vi "Counter Page.vi"(8 "error in (no error)":errorcluster, 11 "Node Ptr":T1 format="%.0x") -> (0 "error out":errorcluster)   [LabVIEW 2020, in "Protection and Counter Addon System Explorer.lvlib"]
uses:
  Protection and Counter Addon System Explorer.lvlib
  <vilib>/NI VeriStand/Custom Device API/Custom Device Item Ref.ctl
  Addon Shared/SubVIs/GUID Lookup.vi
  <vilib>/NI VeriStand/Custom Device API/Custom Device API.lvlib
  SubModules/Frame-Protection-Support/Source/System Explorer/Protection and Counter Support System Explorer.lvlib
  Addon Shared/Protection and Counter Addon Shared.lvlib
panel:
  in  "SHDocVw.IWebBrowser":refnum<k7>(container)
  in  "Rolling Counter Max Count":dbl
  in  "Header":cluster{"Section Name":string}={"Section Name"="Counter Settings"}
  in  "Description":string
  out "Name":string
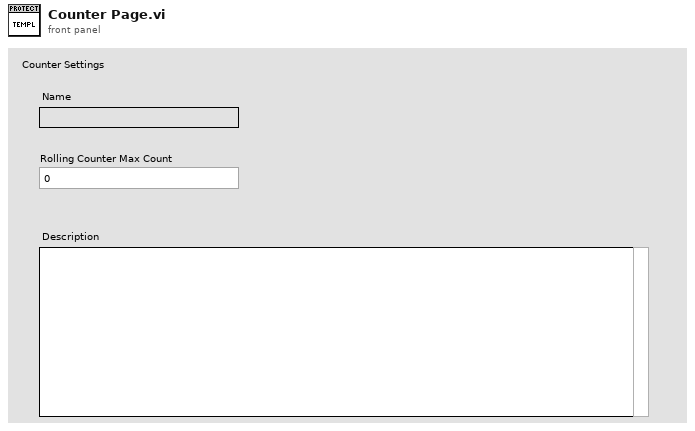
[diagram p1: front panel]
types:
  T1 = typedef "Custom Device API.lvlib/Custom Device Item Ref.ctl" = u64
  T2 = typedef "Custom Device API.lvlib/Custom Device Item Info.ctl" = cluster{"Name":string, "Is Channel":bool, "GUID":string, "Is Waveform":bool}
  T3 = typedef "Custom Device API.lvlib/Custom Device Commands.ctl" = enum16{"Default", "Item renamed", "Shutdown", "Dynamic button pressed"}
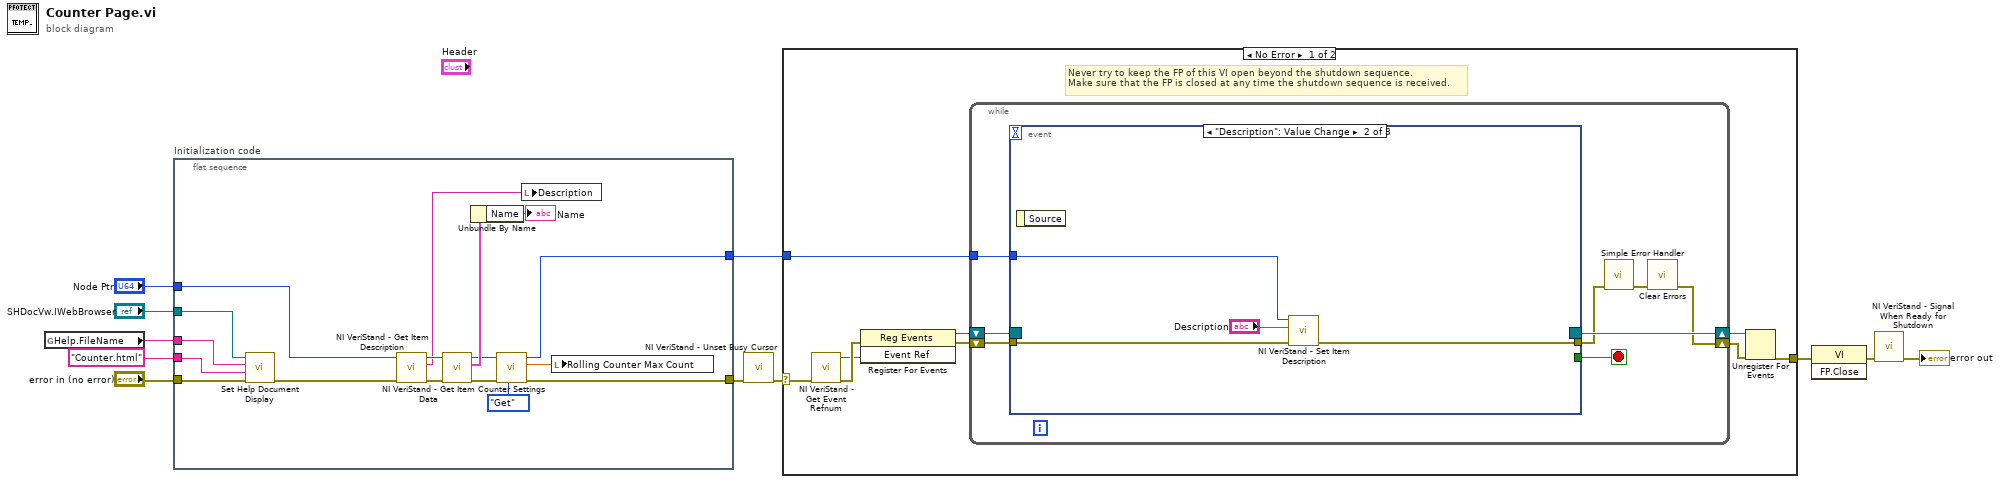
[diagram p0: block diagram]
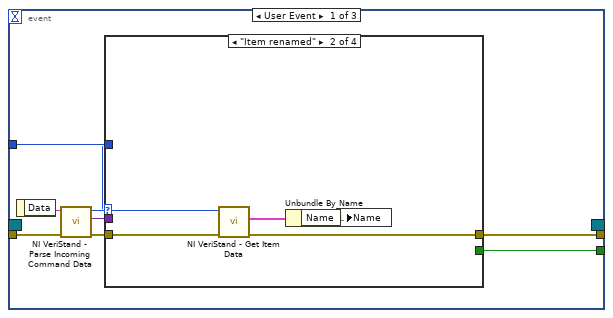
[diagram p2: hidden frame]
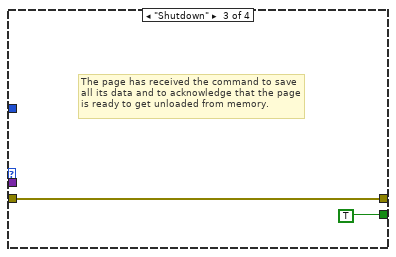
[diagram p4: hidden frame]
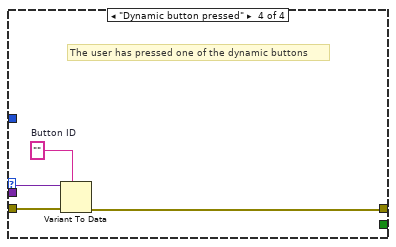
[diagram p5: hidden frame]
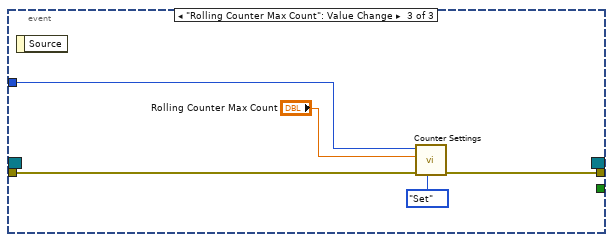
[diagram p6: hidden frame]
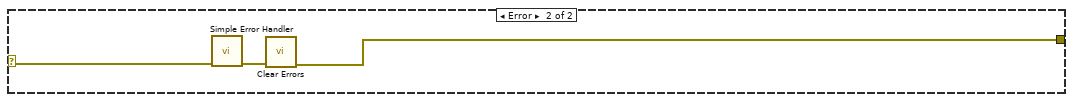
[diagram p7: hidden frame]
diagram:
  n1 = global read "GUID Lookup.vi" "Help.FileName"() -> (w1:string)
  n2 = flat-sequence "Initialization code" {
    tunnel: "error in (no error)" -> [w17]
    tunnel: "Node Ptr" -> [w27]
    tunnel: [w22] -> w7
    tunnel: [w19] -> w4
    tunnel: "Counter.html" ("HTML File") -> [w15]
    tunnel: w1 -> [w14]
    tunnel: "SHDocVw.IWebBrowser" -> [w13]
    frame #0 {
      n3 = call "Set Help Document Display.vi"("error in (no error)"=w17, "HTML File"=w15, "Main CHM File"=w14, "SHDocVw.IWebBrowser2"=w13) -> ("error out"=w16:errorcluster)  [unwired: 7 in]
      n4 = call <vilib>:"NI VeriStand - Get Item Description.vi"("error in (no error)"=w16, "Item Ref in"=w27) -> ("error out"=w25:errorcluster, "Description"=w26:string, "Item Ref out"=w28:T1)  [unwired: 7 out]
      n5 = call <vilib>:"NI VeriStand - Get Item Data.vi"("error in (no error)"=w25, "Item Ref in"=w28) -> ("error out"=w20:errorcluster, "Item Info"=w24:T2, "Item Ref out"=w18:T1)  [unwired: 7 out]
      n6 = Unbundle By Name(w24) -> ("Name"=→"Name":string)
      n7 = call "Counter Settings.vi"("Action"=enum8{"Get", "Set"}."Get", "error in"=w20, "Parent Ref"=w18) -> ("error out"=w22:errorcluster, "Max Count"=w21:dbl, "Parent Ref Out"=w19:T1)  [unwired: 6 in]
      n8 = local write "Description"(w26) -> ()
      n9 = local write "Rolling Counter Max Count"(w21) -> ()
    }
  }
  n10 = call <vilib>:"NI VeriStand - Unset Busy Cursor.vi"("error in (no error)"=w7) -> ("error out"=w6:errorcluster)  [unwired: 10 out]
  n11 = case shown="No Error" w6 {
    selector: w6 -> [w29 w77]
    tunnel: [w34 w75] -> w11
    tunnel: w4 -> [w30 _]
    frame No Error {
      # "Never try to keep the FP of this VI open beyond the shutdown sequence.\nMake sure that the FP is closed at any time the shutdown sequence is received."
      n12 = call <vilib>:"NI VeriStand - Get Event Refnum.vi"("error in (no error)"=w29) -> ("error out"=w37:errorcluster, "Event Ref"=w33:refnum<user-event>)  [unwired: 9 out]
      n13 = register-events(error in=w37, w33) -> (reference out=w31:refnum<event-registration>, error out=w32:errorcluster)  [unwired: 1 in]
      n14 = while {
        tunnel: w30 -> [w41]
        shift-right: [w38] -> w35
        shift-left: w32 -> [w44]
        shift-right: [w45] -> w36
        shift-left: w31 -> [w43]
        stop <- w42 stop-if-true
        n15 = event shown="[1] \"Description\": Value Change" {
          selector: w43 -> [_ _ _]
          dyn-events: [_ _ _] -> w45
          timeout: _ -> [_ _ _]
          tunnel: w44 -> [w53 w68 w74]
          tunnel: [w49 _ _] -> w42
          tunnel: [w48 w67 w72] -> w40
          tunnel: w41 -> [w47 w69 w73]
          event User Event {
            n16 = event-data() -> ("Data"=w52:string)  [unwired: 1 out]
            n17 = call <vilib>:"NI VeriStand - Parse Incoming Command Data.vi"("error in (no error)"=w53, "Incoming data"=w52) -> ("error out"=w51:errorcluster, "Outgoing data"=w46:variant, "Action"=w50:T3)  [unwired: 7 out]
            n18 = case shown="\"Item renamed\"" w50 {
              tunnel: w51 -> [w54 w59 w60 w65]
              tunnel: [_ _ TRUE _] -> w49
              tunnel: [w54 w56 w60 w62] -> w48
              tunnel: w47 -> [_ w58 _ _]
              tunnel: w46 -> [_ _ _ w64]
              frame "Default", Default {
              }
              frame "Item renamed" {
                n19 = call <vilib>:"NI VeriStand - Get Item Data.vi"("error in (no error)"=w59, "Item Ref in"=w58) -> ("error out"=w56:errorcluster, "Item Info"=w57:T2)  [unwired: 8 out]
                n20 = Unbundle By Name(w57) -> ("Name"=w55:string)
                n21 = local write "Name"(w55) -> ()
              }
              frame "Shutdown" {
                # "The page has received the command to save all its data and to acknowledge that the page is ready to get unloaded from memory."
              }
              frame "Dynamic button pressed" {
                w63 = ""  # Button ID
                # "The user has pressed one of the dynamic buttons"
                n22 = Variant To Data(error in=w65, type=w63, Variant=w64) -> (error out=w62:errorcluster)  [unwired: 1 out]
              }
            }
          }
          event "Description": Value Change {
            n23 = event-data() -> ()  [unwired: 2 out]
            n24 = call <vilib>:"NI VeriStand - Set Item Description.vi"("error in (no error)"=w68, "Description"="Description", "Item Ref in"=w69) -> ("error out"=w67:errorcluster)  [unwired: 8 out]
          }
          event "Rolling Counter Max Count": Value Change {
            n25 = event-data() -> ()  [unwired: 2 out]
            n26 = call "Counter Settings.vi"("Action"=enum8{"Get", "Set"}."Set", "error in"=w74, "Max Count"="Rolling Counter Max Count", "Parent Ref"=w73) -> ("error out"=w72:errorcluster)  [unwired: 5 in, 2 out]
          }
        }
        n27 = call <vilib>:"Simple Error Handler.vi"("error in (no error)"=w40) -> ("error out"=w39:errorcluster)  [unwired: 1 in, 7 out]
        n28 = call <vilib>:"Clear Errors.vi"("error in (no error)"=w39) -> ("error out"=w38:errorcluster)  [unwired: 1 in, 5 out]
      }
      n29 = Unregister For Events(event registration refnum=w36, error in=w35) -> (error out=w34:errorcluster)
    }
    frame Error {
      n30 = call <vilib>:"Simple Error Handler.vi"("error in (no error)"=w77) -> ("error out"=w76:errorcluster)  [unwired: 1 in, 7 out]
      n31 = call <vilib>:"Clear Errors.vi"("error in (no error)"=w76) -> ("error out"=w75:errorcluster)  [unwired: 1 in, 5 out]
    }
  }
  n32 = invoke class="VI" method="FP.Close"(error in=w11) -> (error out=w10:errorcluster)  [unwired: 2 in, 2 out]
  n33 = call <vilib>:"NI VeriStand - Signal When Ready for Shutdown.vi"("error in (no error)"=w10) -> ("error out"=→"error out":errorcluster)  [unwired: 10 out]
